vi "PercentToDegrees.vi"(1 "Percent":dbl) -> (0 "Degrees":dbl)   [LabVIEW 2019, in "Zen Analytics.lvlib" / "Zen Analytics.lvclass"]
uses:
  Zen Analytics.lvclass
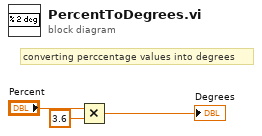
[diagram p0: block diagram]
diagram:
  # "converting perccentage values into degrees"
  n1 = Multiply(x="Percent", y=3.6) -> (x*y=→"Degrees":dbl)
